vi "Map Iteration to Color.vi"(10 "Iteration":u16, 11 "Color Table":u32[](array[numeric])) -> (3 "element":u32)   [LabVIEW 2015]
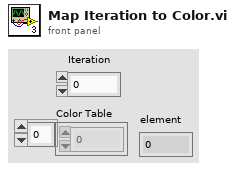
[diagram p1: front panel]
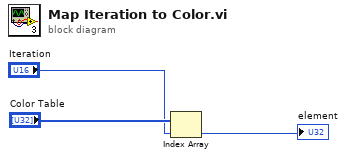
[diagram p0: block diagram]
diagram:
  n1 = Index Array(array="Color Table", index="Iteration") -> (element=→"element":u32)
